vi "sub Make Display.vi"(1 "String5":string, 2 "Decimal Point":enum16{"1", "10", "100", "1000"}(ring)=enum."100", 3 "Number Value":dbl format="%.4f") -> (0 "Fmt Display":cluster{string[], bool, bool, bool, bool})   [LabVIEW 2025]
doc: "Format a number or string for the GUI Demo panel so it looks like the 7-segment displays on the Genesys front panel. Note the GUI shows 5 characters instead of the power supply's 4 characters.\n\nThe decimal point is fixed by the power supply ratings. For example: \n- If the number is 7.40 volts, for a model with a 12-volt rating, set the Decimal Point to 10 and the display shows \"_7.450\".\n- If the number is 7.40 volts, for a model with a 250-volt rating, set the Decimal Point to 100 and the display shows \"_ _7.45\".\n\nIf the String5 string control is *not* blank, the string will show instead of the number. This is useful to show \"OFF\" or faults (\"OVP\" or \"AC\" etc)."
panel:
  # "Format Number or String\nfor 5-Char 7-Segment Display"
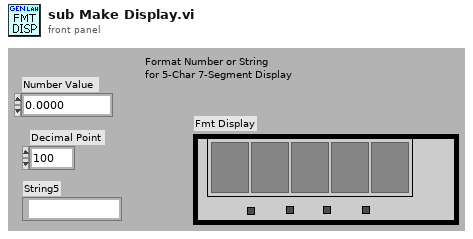
[diagram p1: front panel]
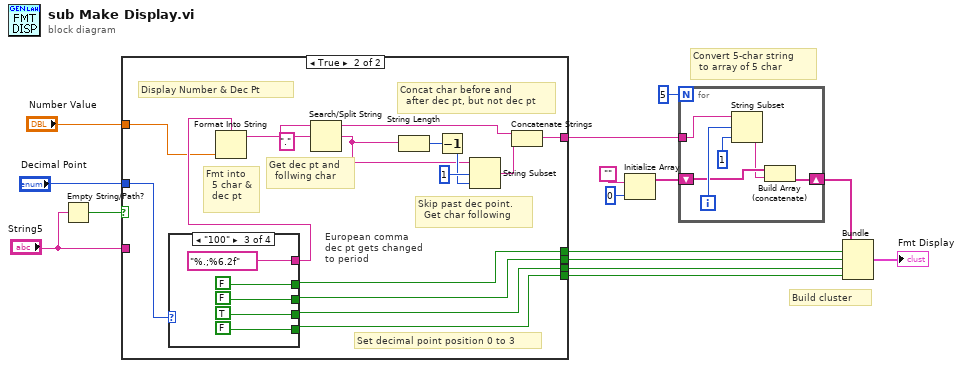
[diagram p0: block diagram]
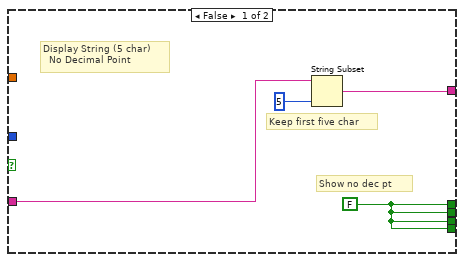
[diagram p2: hidden frame]
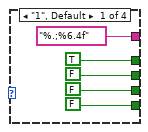
[diagram p3: hidden frame]
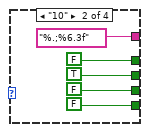
[diagram p4: hidden frame]
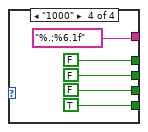
[diagram p5: hidden frame]
diagram:
  # "Build cluster"
  # "Convert 5-char string  \n  to array of 5 char"
  n1 = Empty String/Path?(string/path="String5") -> (empty?=w15:bool)
  n2 = case shown="True" w15 {
    tunnel: "String5" -> [w19 _]
    tunnel: "Decimal Point" -> [_ w35]
    tunnel: "Number Value" -> [_ w33]
    tunnel: [w17 w25] -> w6
    tunnel: [w17 w24] -> w5
    tunnel: [w17 w23] -> w4
    tunnel: [w17 w22] -> w3
    tunnel: [w16 w21] -> w2
    frame False {
      w17 = FALSE
      # "Show no dec pt"
      # "Keep first five char"
      # "Display String (5 char)\n  No Decimal Point"
      n3 = String Subset(string=w19, length (rest)=5 ("length")) -> (substring=w16:string)  [unwired: 1 in]
    }
    frame True {
      # "European comma\ndec pt gets changed\nto period"
      # "Set decimal point position 0 to 3"
      # "Concat char before and  \n  after dec pt, but not dec pt"
      # "Skip past dec point.  \n  Get char following"
      # "Get dec pt and \n  follwing char"
      # "Fmt into\n  5 char & \n  dec pt"
      # "Display Number & Dec Pt"
      n4 = case shown="\"100\"" w35 {
        tunnel: ["%.;%6.4f" "%.;%6.3f" "%.;%6.2f" "%.;%6.1f"] -> w34
        tunnel: [TRUE FALSE FALSE FALSE] -> w25
        tunnel: [FALSE TRUE FALSE FALSE] -> w24
        tunnel: [FALSE FALSE TRUE FALSE] -> w23
        tunnel: [FALSE FALSE FALSE TRUE] -> w22
        frame "1", Default {
        }
        frame "10" {
        }
        frame "100" {
        }
        frame "1000" {
        }
      }
      n5 = Format Into String(format string=w34, w33) -> (resulting string=w27:string)  [unwired: 2 in, 1 out]
      n6 = Search/Split String(string=w27, search string/char (-)="." ("search char (-)")) -> (substring before match=w28:string, match + rest of string=w26:string)  [unwired: 1 in, 1 out]
      n7 = String Length(string=w26) -> (length=w30:i32)
      n8 = Decrement(x=w30) -> (x-1=w29:i32)
      n9 = String Subset(string=w26, offset (0)=1 ("length"), length (rest)=w29) -> (substring=w31:string)
      n10 = Concatenate Strings(w28, w31) -> (w21:string)
    }
  }
  n11 = Initialize Array("", 0) -> (w11:string[])
  n12 = for {
    N: 5 -> [_]
    tunnel: w2 -> [w61]
    shift-right: [w58] -> w10
    shift-left: w11 -> [w57]
    i -> [w59]
    n13 = String Subset(string=w61, offset (0)=w59, length (rest)=1 ("length")) -> (substring=w56:string)
    n14 = Build Array (concatenate)(w57, w56) -> (w58:string[])
  }
  n15 = Bundle(w10, w6, w5, w4, w3) -> (→"Fmt Display":cluster{string[], bool, bool, bool, bool})  [unwired: 1 in]
